vi "Iitialization esp-32 (SubVI).vi"(2 "error in (no error)":errorcluster, 3 "COM-port":refnum<visa-resource-name>) -> (0 "error out":errorcluster, 1 "COM-port out":refnum<visa-resource-name>)   [LabVIEW 2018]
uses:
  <vilib>/Instr/_visa.llb/VISA Configure Serial Port (Instr).vi
panel:
  out "error out 4":errorcluster
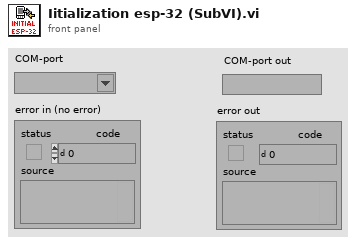
[diagram p1: front panel]
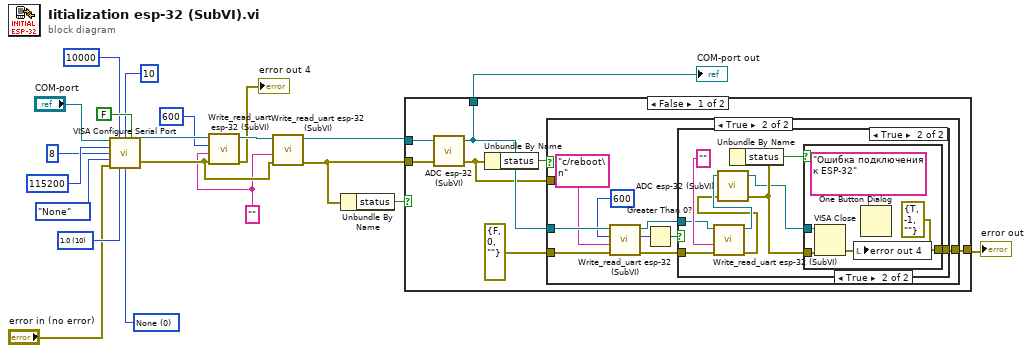
[diagram p0: block diagram]
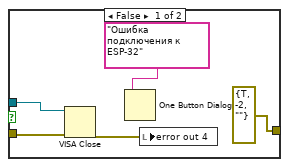
[diagram p3: hidden frame]
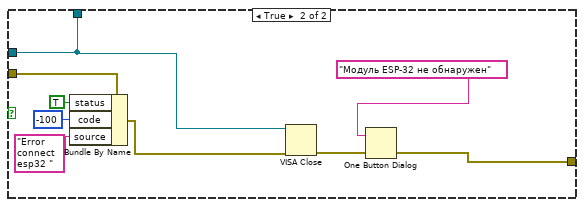
[diagram p5: hidden frame]
diagram:
  w2 = "" ("write buffer")
  w15 = u16 0 items=["None", "XON/XOFF", "RTS/CTS", "XON/XOFF & RTS/CTS", "DTR/DSR", "XON/XOFF & DTR/DSR"] ("flow control (0:none)")
  w16 = u16 10 items=["1.0"=10, "1.5"=15, "2.0"=20] ("stop bits (10: 1 bit)")
  n1 = call-poly "VISA Configure Serial Port"("VISA resource name"="COM-port", "timeout (10sec)"=u32 10000, "termination char\n(0xA = '\\n' = LF)"=u8 10 ("termination char\n(0xA = = LF)"), "Enable Termination\nChar (T)"=FALSE ("Enable Termination\nChar (T)"), "baud rate (9600)"=u32 115200, "data bits (8)"=u16 8, "parity (0:none)"=enum16{"None", "Odd", "Even", "Mark", "Space"}."None", "error in (no error)"="error in (no error)", "stop bits (10: 1 bit)"=w16, "flow control (0:none)"=w15) -> ("VISA resource name out"=w8:refnum<visa-resource-name>, "error out"=w3:errorcluster)  [unwired: 4 in]
  n2 = call "Write_read_uart esp-32 (SubVI).vi"("error in (no error)"=w3, "write buffer"=w2, "milliseconds to wait"=u32 600, "VISA Refnum in"=w8) -> ("error out 4"=→"error out 4":errorcluster, "VISA resource name out"=w4:refnum<visa-resource-name>)  [unwired: 2 out]
  n3 = call "Write_read_uart esp-32 (SubVI).vi"("error in (no error)"=w3, "write buffer"=w2, "VISA Refnum in"=w4) -> ("error out 4"=w6:errorcluster, "VISA resource name out"=w5:refnum<visa-resource-name>)  [unwired: 1 in, 2 out]
  n4 = Unbundle By Name(w6) -> ("status"=w11:bool)
  n5 = case shown="False" w11 {
    tunnel: w6 -> [w28 w62]
    tunnel: w5 -> [w27 w61]
    tunnel: [w24 w59] -> w10
    tunnel: [w26 w61] -> w9
    frame False {
      n6 = call "ADC esp-32 (SubVI).vi"("error in (no error)"=w28, "VISA Refnum in"=w27) -> ("error out"=w23:errorcluster, "VISA resource name out"=w26:refnum<visa-resource-name>)  [unwired: 1 in, 1 out]
      n7 = Unbundle By Name(w23) -> ("status"=w22:bool)
      n8 = case shown="True" w22 {
        tunnel: w26 -> [_ w38]
        tunnel: errorcluster {"status"=FALSE, "code"=0, "source"=""} ("error out") -> [_ w37]
        tunnel: [w29 w30] -> w24
        tunnel: w23 -> [w29 _]
        frame False {
        }
        frame True {
          n9 = call "Write_read_uart esp-32 (SubVI).vi"("error in (no error)"=w37, "write buffer"="c/reboot\n", "milliseconds to wait"=u32 600, "VISA Refnum in"=w38) -> ("error out 4"=w31:errorcluster, "read bite"=w34:u32, "VISA resource name out"=w32:refnum<visa-resource-name>)  [unwired: 1 out]
          n10 = Greater Than 0?(x=w34) -> (x > 0?=w33:bool)
          n11 = case shown="True" w33 {
            tunnel: w32 -> [w42 w51]
            tunnel: w31 -> [w41 w50]
            tunnel: [errorcluster {"status"=TRUE, "code"=-2, "source"=""} ("error out") w47] -> w30
            frame False {
              n12 = VISA Close(VISA resource name=w42, error in (no error)=w41) -> (error out=w39:errorcluster)
              n13 = One Button Dialog(message="Ошибка подключения к ESP-32") -> ()  [unwired: 1 in, 1 out]
              n14 = local write "error out 4"(w39) -> ()
            }
            frame True {
              n15 = call "Write_read_uart esp-32 (SubVI).vi"("error in (no error)"=w50, "write buffer"="", "VISA Refnum in"=w51) -> ("error out 4"=w48:errorcluster, "VISA resource name out"=w49:refnum<visa-resource-name>)  [unwired: 1 in, 2 out]
              n16 = call "ADC esp-32 (SubVI).vi"("error in (no error)"=w48, "VISA Refnum in"=w49) -> ("error out"=w45:errorcluster, "VISA resource name out"=w44:refnum<visa-resource-name>)  [unwired: 1 in, 1 out]
              n17 = Unbundle By Name(w45) -> ("status"=w46:bool)
              n18 = case shown="True" w46 {
                tunnel: [w53 errorcluster {"status"=TRUE, "code"=-1, "source"=""} ("error out")] -> w47
                tunnel: w45 -> [w53 w57]
                tunnel: w44 -> [_ w56]
                frame False {
                }
                frame True {
                  n19 = VISA Close(VISA resource name=w56, error in (no error)=w57) -> (error out=w54:errorcluster)
                  n20 = local write "error out 4"(w54) -> ()
                  n21 = One Button Dialog(message="Ошибка подключения к ESP-32") -> ()  [unwired: 1 in, 1 out]
                }
              }
            }
          }
        }
      }
    }
    frame True {
      n22 = Bundle By Name(cluster=w62, "status"=TRUE, "code"=-100, "source"="Error connect esp32 ") -> (w60:errorcluster)
      n23 = VISA Close(VISA resource name=w61, error in (no error)=w60) -> (error out=w59:errorcluster)
      n24 = One Button Dialog(message="Модуль ESP-32 не обнаружен") -> ()  [unwired: 1 in, 1 out]
    }
  }
  "COM-port out" <- w9
  "error out" <- w10
